vi "Assignment 2.vi"() -> ()   [LabVIEW 2024]
panel:
  in  "Stop":bool
  out "Washing Done":bool
  out "Screen":string="Start the machine"
  in  "Start":bool
  out "Final Spin":bool
  out "Main Wash":bool
  out "Pre-rinse":bool
  in  "Colourful":bool
  in  "Intense":bool
  in  "Quick Wash":bool
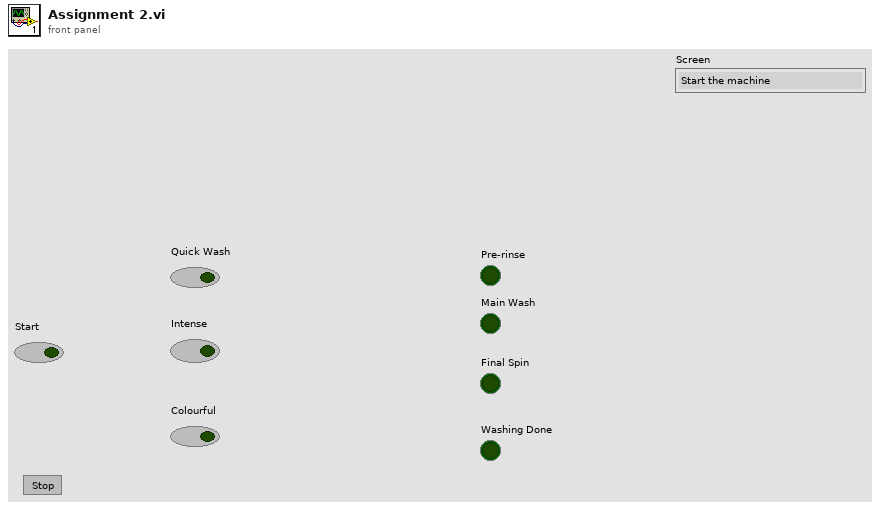
[diagram p1: front panel]
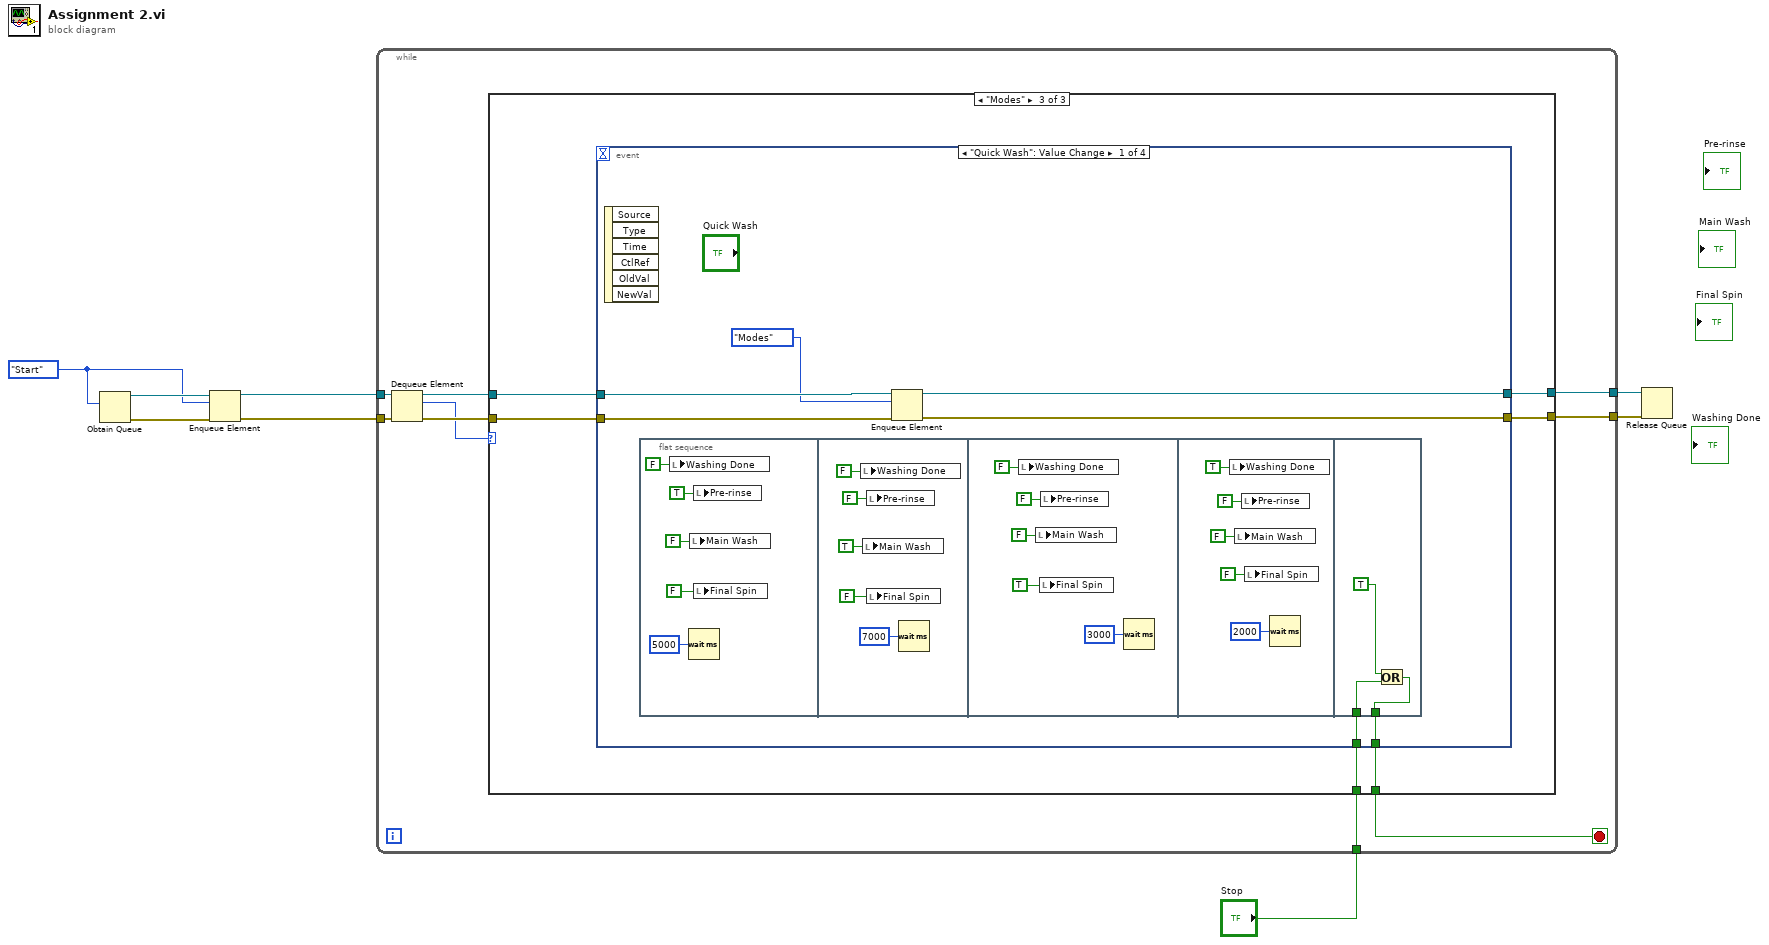
[diagram p0: block diagram]
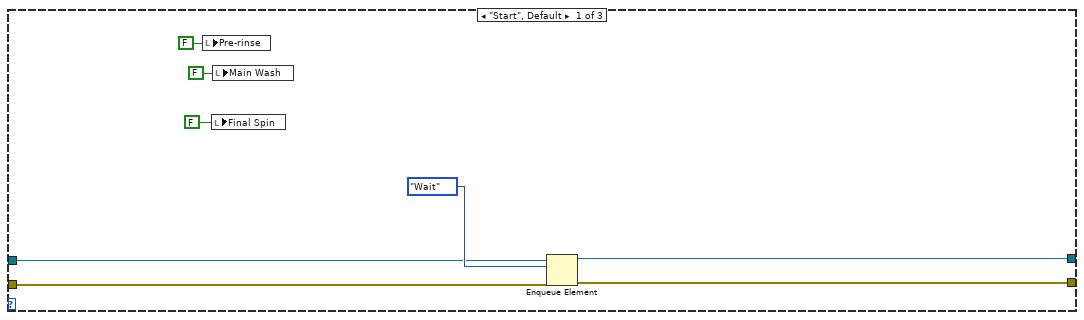
[diagram p2: hidden frame]
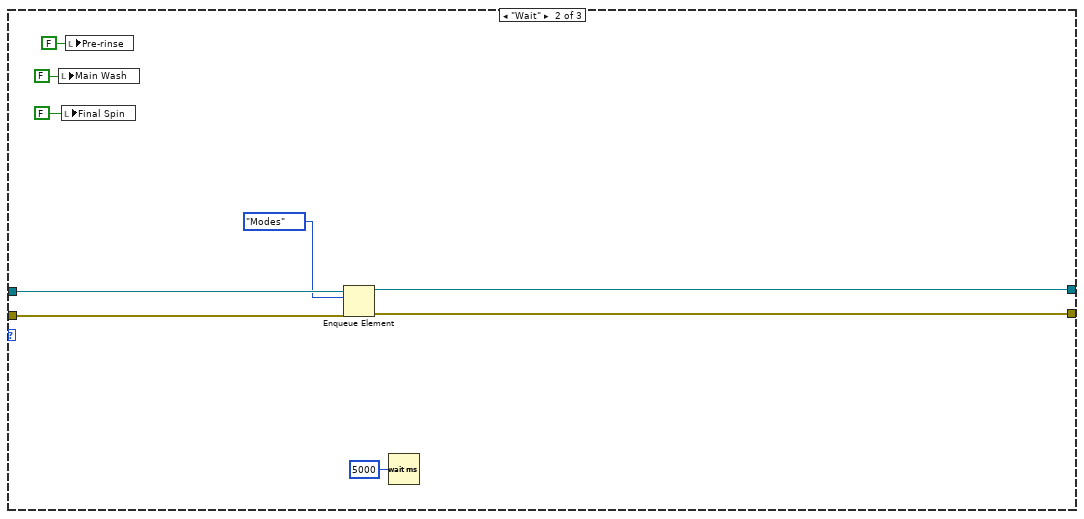
[diagram p3: hidden frame]
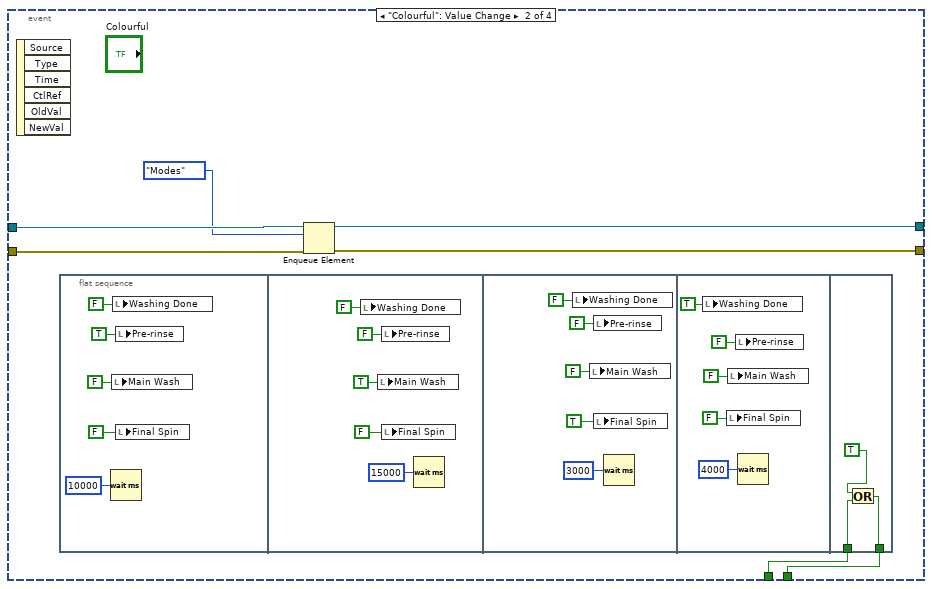
[diagram p4: hidden frame]
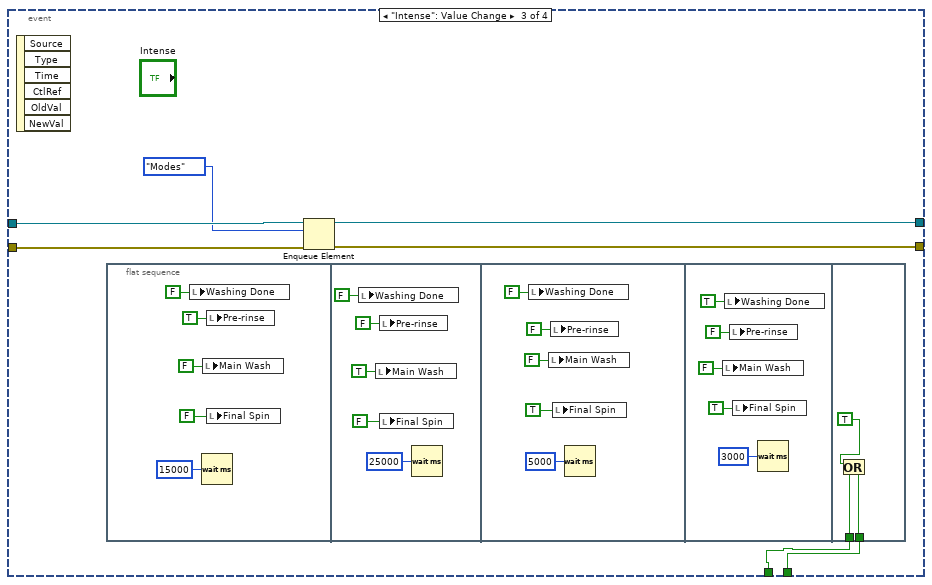
[diagram p5: hidden frame]
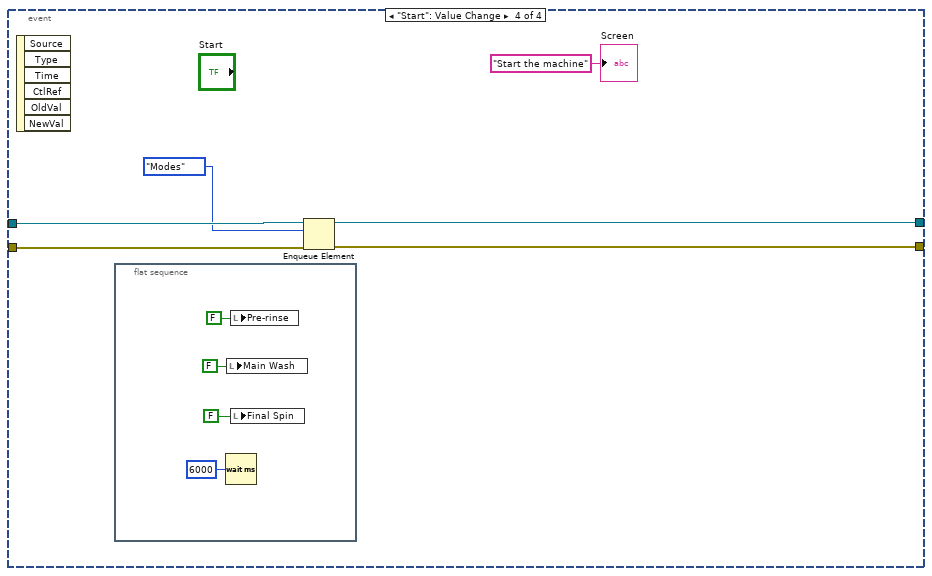
[diagram p6: hidden frame]
diagram:
  w6 = enum16{"Start", "Wait", "Modes"}."Start" ("Enum")
  n1 = Obtain Queue(element data type=w6) -> (queue out=w8:refnum<queue>, error out=w7:errorcluster)  [unwired: 4 in, 1 out]
  n2 = Enqueue Element(queue=w8, element=w6, error in (no error)=w7) -> (queue out=w5:refnum<queue>, error out=w4:errorcluster)  [unwired: 1 in, 1 out]
  n3 = while {
    tunnel: w5 -> [w17]
    tunnel: w4 -> [w16]
    tunnel: [w13] -> w3
    tunnel: [w12] -> w2
    tunnel: "Stop" -> [w9]
    stop <- w10 stop-if-true
    n4 = Dequeue Element(queue=w17, error in (no error)=w16) -> (queue out=w11:refnum<queue>, element=w14:enum16{"Start", "Wait", "Modes"}, error out=w15:errorcluster)  [unwired: 1 in, 1 out]
    n5 = case shown="\"Modes\"" w14 {
      tunnel: w11 -> [w24 w31 w40]
      tunnel: w15 -> [w23 w34 w39]
      tunnel: [w22 w33 w38] -> w13
      tunnel: [w21 w32 w37] -> w12
      tunnel: [_ _ w36] -> w10
      tunnel: w9 -> [_ _ w35]
      frame "Start", Default {
        n6 = local write "Pre-rinse"(FALSE ("Pre-rinse")) -> ()
        n7 = local write "Final Spin"(FALSE ("Final Wash")) -> ()
        n8 = local write "Main Wash"(FALSE ("Main Wash")) -> ()
        n9 = Enqueue Element(queue=w24, element=enum16{"Start", "Wait", "Modes"}."Wait" ("Enum"), error in (no error)=w23) -> (queue out=w22:refnum<queue>, error out=w21:errorcluster)  [unwired: 1 in, 1 out]
      }
      frame "Wait" {
        n10 = local write "Main Wash"(FALSE ("Main Wash")) -> ()
        n11 = local write "Final Spin"(FALSE ("Final Wash")) -> ()
        n12 = local write "Pre-rinse"(FALSE ("Pre-rinse")) -> ()
        n13 = Enqueue Element(queue=w31, element=enum16{"Start", "Wait", "Modes"}."Modes" ("Enum"), error in (no error)=w34) -> (queue out=w33:refnum<queue>, error out=w32:errorcluster)  [unwired: 1 in, 1 out]
        n14 = Wait (ms)(milliseconds to wait=u32 5000) -> ()  [unwired: 1 out]
      }
      frame "Modes" {
        n15 = event shown="[0] \"Quick Wash\": Value Change" {
          selector: _ -> [_ _ _ _]
          dyn-events: _ -> [_ _ _ _]
          timeout: _ -> [_ _ _ _]
          tunnel: w40 -> [w47 w77 w107 w136]
          tunnel: w39 -> [w46 w76 w106 w135]
          tunnel: [w45 w75 w105 w134] -> w38
          tunnel: [w44 w74 w104 w133] -> w37
          tunnel: [w42 w72 w102 _] -> w36
          tunnel: w35 -> [w41 w71 w101 _]
          event "Quick Wash": Value Change {
            n16 = event-data() -> ()  [unwired: 1 in, 6 out]
            n17 = flat-sequence {
              tunnel: [w69] -> w42
              tunnel: w41 -> [w68]
              frame #0 {
                n18 = local write "Washing Done"(FALSE ("Washing Done")) -> ()
                n19 = Wait (ms)(milliseconds to wait=u32 5000) -> ()  [unwired: 1 out]
                n20 = local write "Main Wash"(FALSE ("Main Wash")) -> ()
                n21 = local write "Pre-rinse"(TRUE ("Pre-rinse")) -> ()
                n22 = local write "Final Spin"(FALSE ("Final Wash")) -> ()
              }
              frame #1 {
                n23 = local write "Washing Done"(FALSE ("Washing Done")) -> ()
                n24 = local write "Main Wash"(TRUE ("Main Wash")) -> ()
                n25 = local write "Pre-rinse"(FALSE ("Pre-rinse")) -> ()
                n26 = local write "Final Spin"(FALSE ("Final Wash")) -> ()
                n27 = Wait (ms)(milliseconds to wait=u32 7000) -> ()  [unwired: 1 out]
              }
              frame #2 {
                n28 = local write "Washing Done"(FALSE ("Washing Done")) -> ()
                n29 = local write "Main Wash"(FALSE ("Main Wash")) -> ()
                n30 = local write "Final Spin"(TRUE ("Final Wash")) -> ()
                n31 = local write "Pre-rinse"(FALSE ("Pre-rinse")) -> ()
                n32 = Wait (ms)(milliseconds to wait=u32 3000) -> ()  [unwired: 1 out]
              }
              frame #3 {
                n33 = local write "Washing Done"(TRUE ("Washing Done")) -> ()
                n34 = local write "Main Wash"(FALSE ("Main Wash")) -> ()
                n35 = local write "Pre-rinse"(FALSE ("Pre-rinse")) -> ()
                n36 = local write "Final Spin"(FALSE ("Final Spin")) -> ()
                n37 = Wait (ms)(milliseconds to wait=u32 2000) -> ()  [unwired: 1 out]
              }
              frame #4 {
                n38 = Or(x=TRUE, y=w68) -> (x .or. y?=w69:bool)
              }
            }
            n39 = Enqueue Element(queue=w47, element=enum16{"Start", "Wait", "Modes"}."Modes" ("Enum"), error in (no error)=w46) -> (queue out=w45:refnum<queue>, error out=w44:errorcluster)  [unwired: 1 in, 1 out]
          }
          event "Colourful": Value Change {
            n40 = event-data() -> ()  [unwired: 1 in, 6 out]
            n41 = flat-sequence {
              tunnel: [w99] -> w72
              tunnel: w71 -> [w98]
              frame #0 {
                n42 = Wait (ms)(milliseconds to wait=u32 10000) -> ()  [unwired: 1 out]
                n43 = local write "Main Wash"(FALSE ("Main Wash")) -> ()
                n44 = local write "Washing Done"(FALSE ("Washing Done")) -> ()
                n45 = local write "Pre-rinse"(TRUE ("Pre-rinse")) -> ()
                n46 = local write "Final Spin"(FALSE ("Final Wash")) -> ()
              }
              frame #1 {
                n47 = local write "Washing Done"(FALSE ("Washing Done")) -> ()
                n48 = local write "Main Wash"(TRUE ("Main Wash")) -> ()
                n49 = local write "Pre-rinse"(FALSE ("Pre-rinse")) -> ()
                n50 = local write "Final Spin"(FALSE ("Final Wash")) -> ()
                n51 = Wait (ms)(milliseconds to wait=u32 15000) -> ()  [unwired: 1 out]
              }
              frame #2 {
                n52 = local write "Washing Done"(FALSE ("Washing Done")) -> ()
                n53 = local write "Main Wash"(FALSE ("Main Wash")) -> ()
                n54 = local write "Pre-rinse"(FALSE ("Pre-rinse")) -> ()
                n55 = local write "Final Spin"(TRUE ("Final Wash")) -> ()
                n56 = Wait (ms)(milliseconds to wait=u32 3000) -> ()  [unwired: 1 out]
              }
              frame #3 {
                n57 = local write "Washing Done"(TRUE ("Washing Done")) -> ()
                n58 = local write "Final Spin"(FALSE ("Final Spin")) -> ()
                n59 = local write "Main Wash"(FALSE ("Main Wash")) -> ()
                n60 = local write "Pre-rinse"(FALSE ("Pre-rinse")) -> ()
                n61 = Wait (ms)(milliseconds to wait=u32 4000) -> ()  [unwired: 1 out]
              }
              frame #4 {
                n62 = Or(x=TRUE, y=w98) -> (x .or. y?=w99:bool)
              }
            }
            n63 = Enqueue Element(queue=w77, element=enum16{"Start", "Wait", "Modes"}."Modes" ("Enum"), error in (no error)=w76) -> (queue out=w75:refnum<queue>, error out=w74:errorcluster)  [unwired: 1 in, 1 out]
          }
          event "Intense": Value Change {
            n64 = event-data() -> ()  [unwired: 1 in, 6 out]
            n65 = flat-sequence {
              tunnel: [w129] -> w102
              tunnel: w101 -> [w128]
              frame #0 {
                n66 = local write "Washing Done"(FALSE ("Washing Done")) -> ()
                n67 = Wait (ms)(milliseconds to wait=u32 15000) -> ()  [unwired: 1 out]
                n68 = local write "Main Wash"(FALSE ("Main Wash")) -> ()
                n69 = local write "Pre-rinse"(TRUE ("Pre-rinse")) -> ()
                n70 = local write "Final Spin"(FALSE ("Final Wash")) -> ()
              }
              frame #1 {
                n71 = local write "Washing Done"(FALSE ("Washing Done")) -> ()
                n72 = local write "Main Wash"(TRUE ("Main Wash")) -> ()
                n73 = local write "Pre-rinse"(FALSE ("Pre-rinse")) -> ()
                n74 = local write "Final Spin"(FALSE ("Final Wash")) -> ()
                n75 = Wait (ms)(milliseconds to wait=u32 25000) -> ()  [unwired: 1 out]
              }
              frame #2 {
                n76 = local write "Washing Done"(FALSE ("Washing Done")) -> ()
                n77 = local write "Main Wash"(FALSE ("Main Wash")) -> ()
                n78 = local write "Pre-rinse"(FALSE ("Pre-rinse")) -> ()
                n79 = local write "Final Spin"(TRUE ("Final Wash")) -> ()
                n80 = Wait (ms)(milliseconds to wait=u32 5000) -> ()  [unwired: 1 out]
              }
              frame #3 {
                n81 = local write "Main Wash"(FALSE ("Main Wash")) -> ()
                n82 = local write "Washing Done"(TRUE ("Washing Done")) -> ()
                n83 = local write "Pre-rinse"(FALSE ("Pre-rinse")) -> ()
                n84 = local write "Final Spin"(TRUE ("Final Spin")) -> ()
                n85 = Wait (ms)(milliseconds to wait=u32 3000) -> ()  [unwired: 1 out]
              }
              frame #4 {
                n86 = Or(x=TRUE, y=w128) -> (x .or. y?=w129:bool)
              }
            }
            n87 = Enqueue Element(queue=w107, element=enum16{"Start", "Wait", "Modes"}."Modes" ("Enum"), error in (no error)=w106) -> (queue out=w105:refnum<queue>, error out=w104:errorcluster)  [unwired: 1 in, 1 out]
          }
          event "Start": Value Change {
            n88 = event-data() -> ()  [unwired: 1 in, 6 out]
            n89 = flat-sequence {
              frame #0 {
                n90 = Wait (ms)(milliseconds to wait=u32 6000) -> ()  [unwired: 1 out]
                n91 = local write "Main Wash"(FALSE ("Main Wash")) -> ()
                n92 = local write "Pre-rinse"(FALSE ("Pre-rinse")) -> ()
                n93 = local write "Final Spin"(FALSE ("Final Wash")) -> ()
              }
            }
            n94 = Enqueue Element(queue=w136, element=enum16{"Start", "Wait", "Modes"}."Modes" ("Enum"), error in (no error)=w135) -> (queue out=w134:refnum<queue>, error out=w133:errorcluster)  [unwired: 1 in, 1 out]
            "Screen" <- "Start the machine"
          }
        }
      }
    }
  }
  n95 = Release Queue(queue=w3, error in (no error)=w2) -> ()  [unwired: 1 in, 3 out]
